vi "AspicSettingsDialog.vi"(6 "error in (no error)":errorcluster, 9 "Aspic Seeting In":T1) -> (0 "error out":errorcluster, 2 "UI Refresh Needed?":bool, 3 "Aspic Seeting Out":T1)   [LabVIEW 2014]
uses:
  controls/AspicMode.ctl
  controls/AspicSettings.ctl
panel:
  in  "AF1":bool
  in  "Mode":T2
  in  "RC":u8 format="%b"
  in  "Gain":u8 format="%b"
  in  "Cancel Button":bool
  in  "OK Button":bool
  # "ASPIC settings"
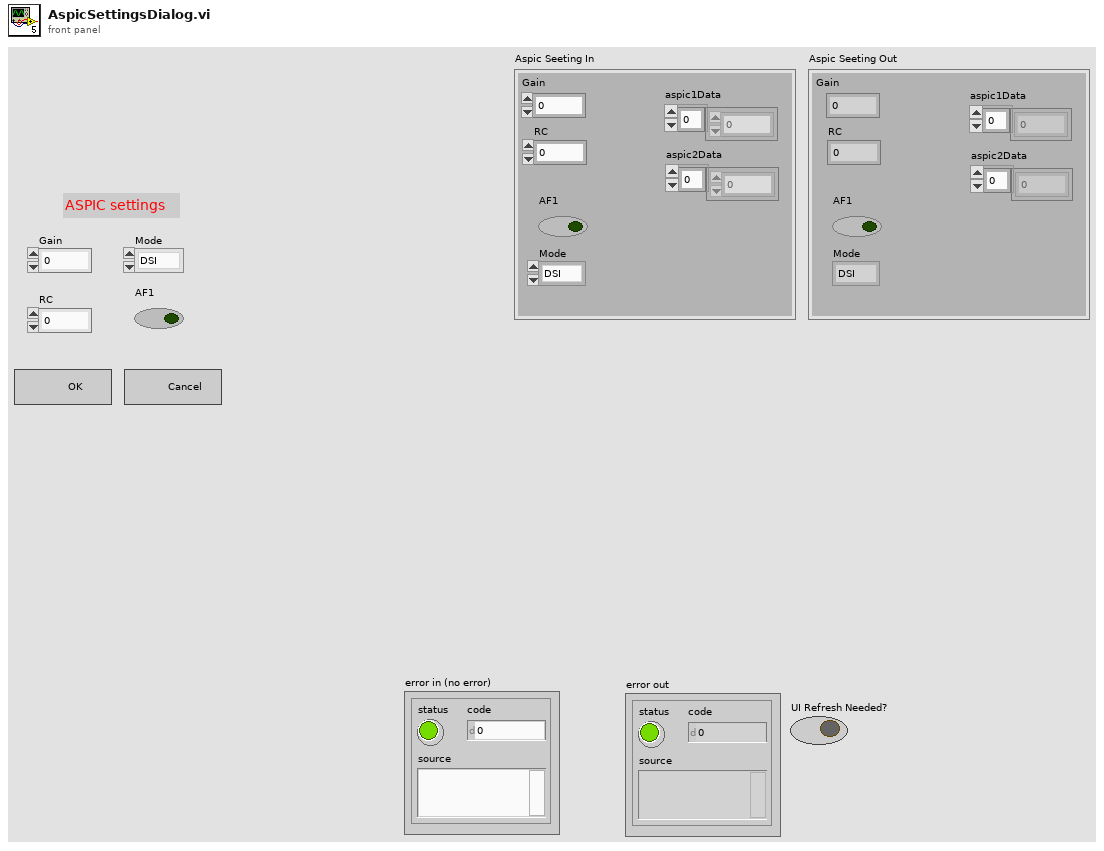
[diagram p1: front panel]
types:
  T1 = typedef "AspicSettings.ctl" = cluster{"Gain":u8, "RC":u8, "aspic1Data":u32[], "aspic2Data":u32[], "AF1":bool, "Mode":T2}
  T2 = typedef "AspicMode.ctl" = enum16{"DSI", "TM"}
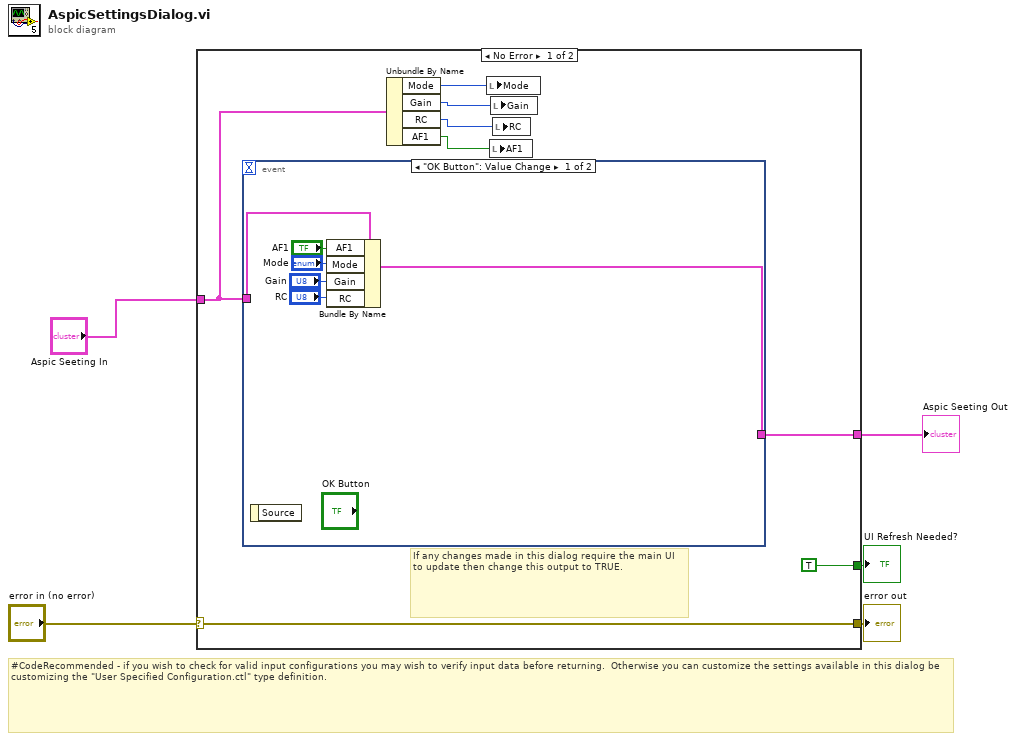
[diagram p0: block diagram]
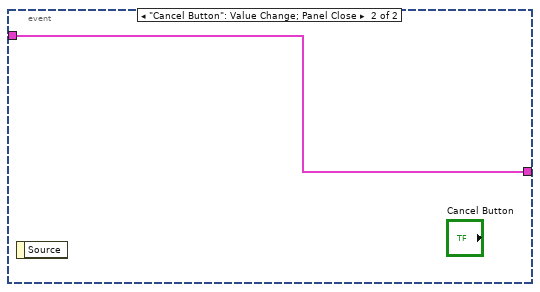
[diagram p2: hidden frame]
diagram:
  # "#CodeRecommended - if you wish to check for valid input configurations you may wish to verify input data before returning.  Otherwise you can customize the settings available in this dialog be customizing the \"User Specified Configuration.ctl\" type definition."
  n1 = case shown="No Error" "error in (no error)" {
    selector: "error in (no error)" -> [w13 w22]
    tunnel: [w13 w22] -> w4
    tunnel: "Aspic Seeting In" -> [w10 w21]
    tunnel: [w12 w21] -> w2
    tunnel: [TRUE ("UI Refresh Needed?") _] -> w3
    frame No Error {
      # "If any changes made in this dialog require the main UI to update then change this output to TRUE."
      n2 = event shown="[0] \"OK Button\": Value Change" {
        selector: _ -> [_ _]
        dyn-events: _ -> [_ _]
        timeout: _ -> [_ _]
        tunnel: [w19 w20] -> w12
        tunnel: w10 -> [w14 w20]
        event "OK Button": Value Change {
          n3 = event-data() -> ()  [unwired: 1 in, 1 out]
          n4 = Bundle By Name(cluster=w14, "AF1"="AF1", "Mode"="Mode", "Gain"="Gain", "RC"="RC") -> (w19:T1)
        }
        event "Cancel Button": Value Change; Panel Close {
          n5 = event-data() -> ()  [unwired: 1 in, 1 out]
        }
      }
      n6 = Unbundle By Name(w10) -> ("Mode"=w9:T2, "Gain"=w8:u8, "RC"=w7:u8, "AF1"=w6:bool)
      n7 = local write "Mode"(w9) -> ()
      n8 = local write "AF1"(w6) -> ()
      n9 = local write "Gain"(w8) -> ()
      n10 = local write "RC"(w7) -> ()
    }
    frame Error {
    }
  }
  "UI Refresh Needed?" <- w3
  "error out" <- w4
  "Aspic Seeting Out" <- w2
